vi "From Byte Array (Characterization Data).vi"(5 "byte array in":u8[](array[numeric]) format="%x", 7 "Device Data Header":T4={"Checksum"=0, "Number of Channels"=0, "Number of Attenuations"=[], "Number of Attenuator Settings"=[], "Number of Gain Settings"=[], "Pointer to Cal Data"=[], "Number of Reserved Bytes"=7, "Number of Frequencies"=[]} {"Checksum" format="%x"}, 9 "channel":i32, 11 "Error In":errorcluster) -> (6 "Characterization Data":T1 {"Frequencies [Hz]" format="%#_6p"}, 15 "Error Out":errorcluster)   [LabVIEW 2013]
uses:
  <instrlib>/ni579x/Config/v1/Shared/Types/EEPROM/ni579x EEPROM Device Data Header.ctl
  <instrlib>/ni579x/Config/v1/Shared/Types/ni579x Characterization Data.ctl
  <instrlib>/ni579x/Config/v1/Shared/Types/ni579x IQ Imbalance.ctl
  <instrlib>/ni579x/Config/v1/Shared/Types/ni579x Gain to Attenuation Mapping.ctl
  <instrlib>/ni579x/Config/v1/Shared/Conversions/From Byte Array (F32).vi
  <instrlib>/ni579x/Config/v1/Shared/Conversions/From Byte Array (U8).vi
  <instrlib>/ni579x/Config/v1/Shared/Conversions/From Byte Array (U16).vi
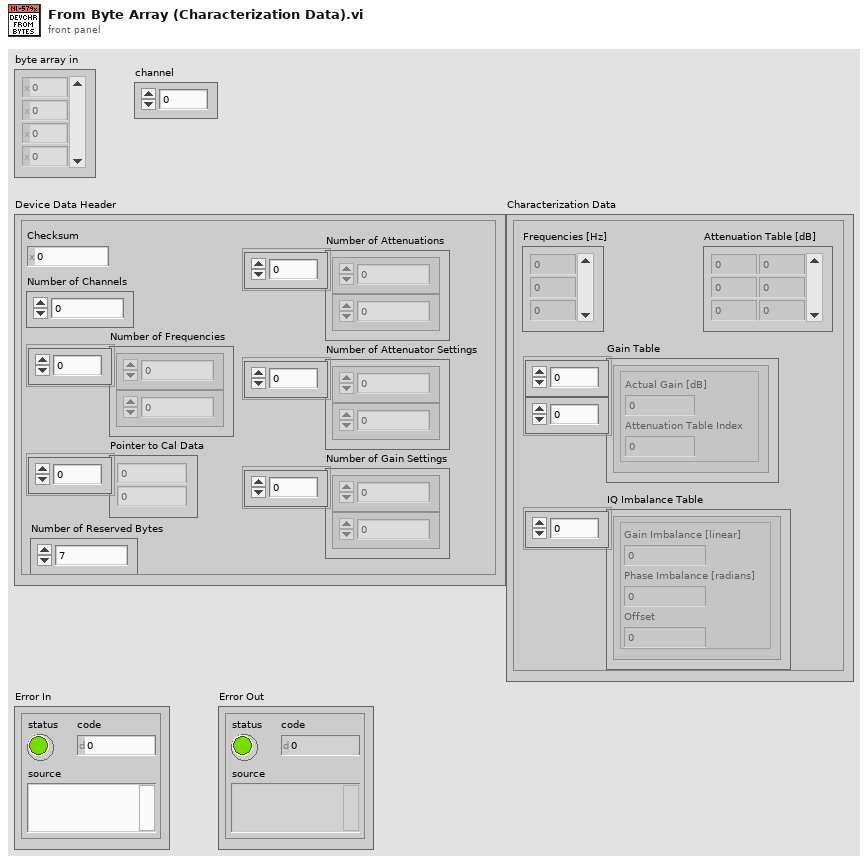
[diagram p1: front panel]
types:
  T1 = typedef "ni579x Characterization Data.ctl" = cluster{"Attenuation Table [dB]":dbl[][], "Frequencies [Hz]":dbl[], "IQ Imbalance Table":T2[], "Gain Table":T3[][]}
  T2 = typedef "ni579x IQ Imbalance.ctl" = cluster{"Gain Imbalance [linear]":dbl, "Phase Imbalance [radians]":dbl, "Offset":cdb}
  T3 = typedef "ni579x Gain to Attenuation Mapping.ctl" = cluster{"Actual Gain [dB]":dbl, "Attenuation Table Index":i32}
  T4 = typedef "ni579x EEPROM Device Data Header.ctl" = cluster{"Checksum":u32, "Number of Channels":u8, "Number of Attenuations":u16[], "Number of Attenuator Settings":u8[], "Number of Gain Settings":u8[], "Pointer to Cal Data":u32[], "Number of Reserved Bytes":i32, "Number of Frequencies":u16[]}
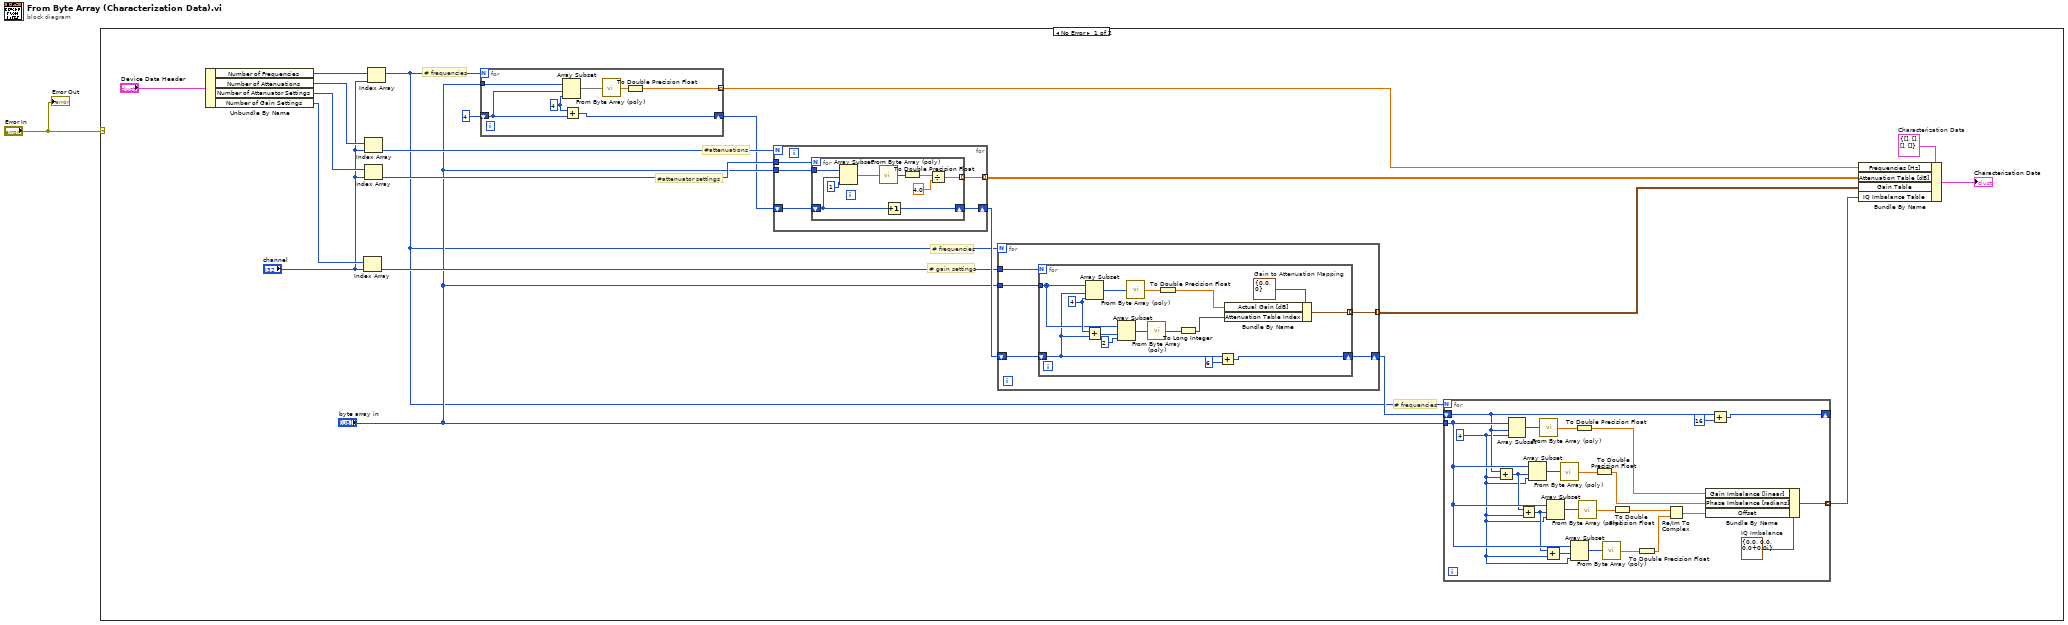
[diagram p0: block diagram]
diagram:
  n1 = case shown="No Error" "Error In" {
    frame No Error {
      w20 = T1 {"Attenuation Table [dB]"=[], "Frequencies [Hz]"=[], "IQ Imbalance Table"=[], "Gain Table"=[]}  # Characterization Data
      # "# gain settings"
      # "#attenuator settings"
      # "#attenuations"
      # "# frequencies"
      # "# frequencies"
      # "# frequencies"
      n2 = Unbundle By Name("Device Data Header") -> ("Number of Frequencies"=w21:u16[], "Number of Attenuations"=w14:u16[], "Number of Attenuator Settings"=w12:u8[], "Number of Gain Settings"=w10:u8[])
      n3 = Index Array(array=w10, index="channel") -> (element=w9:u8)
      n4 = Index Array(array=w12, index="channel") -> (element=w11:u8)
      n5 = Index Array(array=w14, index="channel") -> (element=w13:u16)
      n6 = Index Array(array=w21, index="channel") -> (element=w4:u16)
      n7 = for {
        N: w4 -> [_]
        tunnel: "byte array in" -> [w27]
        shift-right: [w23] -> w3
        shift-left: 4 -> [w26]
        tunnel: [w25] -> w2 mode=indexing
        w24 = 4 ("length")
        n8 = Array Subset(array=w27, index=w26, length=w24) -> (w28:u8[])
        n9 = Add(x=w24, y=w26) -> (x+y=w23:i32)
        n10 = call-poly <instrlib>:"From Byte Array (poly).vi"("byte array in"=w28) -> ("element out"=w29:sgl)
        n11 = To Double Precision Float(number=w29) -> (double precision float=w25:dbl)
      }
      n12 = for {
        N: w13 -> [_]
        tunnel: w11 -> [w77]
        tunnel: "byte array in" -> [w76]
        shift-right: [w73] -> w16
        shift-left: w3 -> [w75]
        tunnel: [w74] -> w17 mode=indexing
        n13 = for {
          N: w77 -> [_]
          tunnel: w76 -> [w86]
          shift-right: [w82] -> w73
          shift-left: w75 -> [w83]
          tunnel: [w78] -> w74 mode=indexing
          n14 = Array Subset(array=w86, index=w83, length=1) -> (w84:u8[])
          n15 = call-poly <instrlib>:"From Byte Array (poly).vi"("byte array in"=w84) -> ("element out"=w81:u8)
          n16 = Increment(x=w83) -> (x+1=w82:i32)
          n17 = To Double Precision Float(number=w81) -> (double precision float=w80:dbl)
          n18 = Divide(x=w80, y=4.0) -> (x/y=w78:dbl)
        }
      }
      n19 = for {
        N: w4 -> [_]
        tunnel: w9 -> [w57]
        tunnel: [w56] -> w19 mode=indexing
        shift-right: [w53] -> w15
        shift-left: w16 -> [w55]
        tunnel: "byte array in" -> [w54]
        n20 = for {
          N: w57 -> [_]
          tunnel: [w71] -> w56 mode=indexing
          shift-right: [w58] -> w53
          shift-left: w55 -> [w60]
          tunnel: w54 -> [w63]
          w68 = 4 ("length")
          w72 = T3 {"Actual Gain [dB]"=0.0, "Attenuation Table Index"=0}  # Gain to Attenuation Mapping
          n21 = Array Subset(array=w63, index=w60, length=w68) -> (w69:u8[])
          n22 = Add(x=w68, y=w60) -> (x+y=w67:i32)
          n23 = Array Subset(array=w63, index=w67, length=2) -> (w64:u8[])
          n24 = call-poly <instrlib>:"From Byte Array (poly).vi"("byte array in"=w69) -> ("element out"=w66:sgl)
          n25 = call-poly <instrlib>:"From Byte Array (poly).vi"("byte array in"=w64) -> ("element out"=w62:u16)
          n26 = To Double Precision Float(number=w66) -> (double precision float=w65:dbl)
          n27 = To Long Integer(number=w62) -> (32bit integer=w61:i32)
          n28 = Add(x=w60, y=6) -> (x+y=w58:i32)
          n29 = Bundle By Name(cluster=w72, "Actual Gain [dB]"=w65, "Attenuation Table Index"=w61) -> (w71:T3)
        }
      }
      n30 = for {
        N: w4 -> [_]
        tunnel: [w51] -> w18 mode=indexing
        shift-right: [w31] -> _
        shift-left: w15 -> [w33]
        tunnel: "byte array in" -> [w41]
        w30 = 4 ("length")
        w52 = T2 {"Gain Imbalance [linear]"=0.0, "Phase Imbalance [radians]"=0.0, "Offset"=0.0+0.0i}  # IQ Imbalance
        n31 = Add(x=w33, y=w30) -> (x+y=w40:i32)
        n32 = Array Subset(array=w41, index=w33, length=w30) -> (w50:u8[])
        n33 = Add(x=w40, y=w30) -> (x+y=w39:i32)
        n34 = Array Subset(array=w41, index=w40, length=w30) -> (w47:u8[])
        n35 = call-poly <instrlib>:"From Byte Array (poly).vi"("byte array in"=w50) -> ("element out"=w49:sgl)
        n36 = Add(x=w39, y=w30) -> (x+y=w42:i32)
        n37 = Array Subset(array=w41, index=w39, length=w30) -> (w46:u8[])
        n38 = call-poly <instrlib>:"From Byte Array (poly).vi"("byte array in"=w47) -> ("element out"=w48:sgl)
        n39 = Array Subset(array=w41, index=w42, length=w30) -> (w43:u8[])
        n40 = To Double Precision Float(number=w49) -> (double precision float=w34:dbl)
        n41 = call-poly <instrlib>:"From Byte Array (poly).vi"("byte array in"=w46) -> ("element out"=w45:sgl)
        n42 = To Double Precision Float(number=w48) -> (double precision float=w35:dbl)
        n43 = call-poly <instrlib>:"From Byte Array (poly).vi"("byte array in"=w43) -> ("element out"=w44:sgl)
        n44 = To Double Precision Float(number=w45) -> (double precision float=w38:dbl)
        n45 = To Double Precision Float(number=w44) -> (double precision float=w37:dbl)
        n46 = Re/Im To Complex(1:w37, 2:w38) -> (0:w36:cdb)
        n47 = Bundle By Name(cluster=w52, "Gain Imbalance [linear]"=w34, "Phase Imbalance [radians]"=w35, "Offset"=w36) -> (w51:T2)
        n48 = Add(x=w33, y=16) -> (x+y=w31:i32)
      }
      n49 = Bundle By Name(cluster=w20, "Frequencies [Hz]"=w2, "Attenuation Table [dB]"=w17, "Gain Table"=w19, "IQ Imbalance Table"=w18) -> (→"Characterization Data":T1)
    }
    frame Error {
    }
  }
  "Error Out" <- "Error In"
